vi "Teleop.vi"(10 "Match Info":T1={"Autonomous Elapsed Seconds"=0.0, "TeleOp Elapsed Seconds"=0.0, "Disabled Elapsed Seconds"=0.0, "Visited Autonomous"=FALSE, "Visited TeleOp"=FALSE, "Visited Disabled"=FALSE, "Autonomous Settings"={"Autonomous Style"=enum."Independent", "VI Refnum"=refnum}}, 11 "Call Context":T2) -> ()   [LabVIEW 2015]
doc: "This VI is called for each TeleOp packet received from the DS where the robot is not disabled. It is often used to read from the joysticks and update I/O or to update setpoints for timed control loops. It should complete and return within 20 milliseconds or it may miss DS packets."
uses:
  <vilib>/Rock Robotics/WPI/DriverStation/WPI_DriverStationDerivedRobotMode.ctl
  <vilib>/Rock Robotics/WPI/DriverStation/WPI_DriverStationMatch Info.ctl
  <vilib>/Rock Robotics/WPI/Utilities/WPI_GetSetVariantRefNum.vi
  <vilib>/Rock Robotics/Network Tables/NT Write Boolean Array.vi
  <vilib>/Rock Robotics/Network Tables/NT Write Numeric Array.vi
  <vilib>/Rock Robotics/Network Tables/NT Read Boolean.vi
  <vilib>/Rock Robotics/Network Tables/NT Read Number.vi
  <vilib>/Rock Robotics/Network Tables/NT Write Number.vi
  <vilib>/Rock Robotics/Network Tables/NT Write Boolean.vi
panel:
  out "Sample Slider 0":dbl(slide) scale=0.0..5.0
  out "Sample Boolean 1":bool
  out "Sample Boolean 0":bool
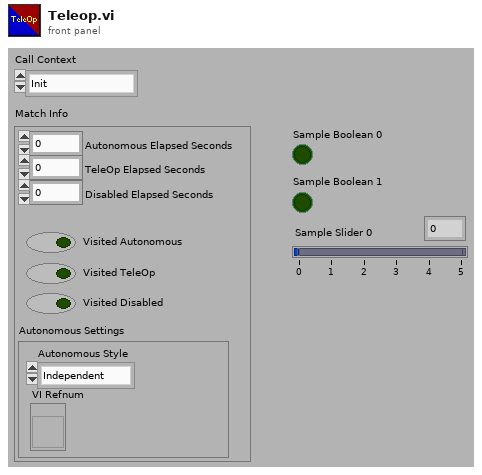
[diagram p1: front panel]
types:
  T1 = typedef "WPI_DriverStationMatch Info.ctl" = cluster{"Autonomous Elapsed Seconds":dbl, "TeleOp Elapsed Seconds":dbl, "Disabled Elapsed Seconds":dbl, "Visited Autonomous":bool, "Visited TeleOp":bool, "Visited Disabled":bool, "Autonomous Settings":cluster{"Autonomous Style":enum16{"Iterative", "Independent"}, "VI Refnum":refnum<vi>}}
  T2 = typedef "WPI_DriverStationDerivedRobotMode.ctl" = enum16{"Init", "Execute", "Stop"}
  T3 = typedef "WPI_MotorControlDeviceRef.ctl" = cluster{"DeviceStatus":errorcluster, "Type":T4, "PWM":cluster{"PWM Channel":T5, "DeadBand":T6}, "CAN":cluster{"Device Number":u8, "Control Mode":T7, "Semaphore":T8, "Max Vout":dbl, "TalonSRX Control Mode":T9}, "Invert":bool}
  T4 = typedef "WPI_MotorControlType.ctl" = enum16{"PWM", "CAN", "CANTalonSRX"}
  T5 = typedef "FPGA_DIOPWMChannel.ctl" = enum8{"PWM 0", "PWM 1", "PWM 2", "PWM 3", "PWM 4", "PWM 5", "PWM 6", "PWM 7", "PWM 8", "PWM 9", "PWM MXP 0", "PWM MXP 1", "PWM MXP 2", "PWM MXP 3", "PWM MXP 4", "PWM MXP 5", "PWM MXP 6", "PWM MXP 7", "PWM MXP 8", "PWM MXP 9", "Invalid"}
  T6 = typedef "WPI_PWMDeadband.ctl" = cluster{"Name":string, "maxPositivePwm":i32, "minPositivePwm":i32, "centerPwm":i32, "maxNegativePwm":i32, "minNegativePwm":i32, "angularRange":u16}
  T7 = typedef "WPI_CANJaguar_ControlMode.ctl" = enum8{"Percent VBus", "Current", "Speed", "Position", "Voltage"}
  T8 = typedef "Semaphore RefNum" = refnum<k1>
  T9 = typedef "WPI_CANTalonSRX_APIControlMode.ctl" = enum8{"Percent VBus", "Speed", "Position", "Slave", "Unchanged / Invalid", "Voltage Compensation", "Current", "Motion Profile"}
  T10 = typedef "WPI_RobotDriveDevRef.ctl" = cluster{"DevStatus":errorcluster, "Motors[]":T3[], "Square Inputs":bool, "Max Output":dbl}
  T11 = typedef "WPI_JoystickDevRef.ctl" = cluster{"Device":T12}
  T12 = typedef "WPI_JoystickDeviceEnum.ctl" = enum16{"USB 0", "USB 1", "USB 2", "USB 3", "USB 4", "USB 5"}
  T13 = typedef "WPI_DigitalInputDevRef.ctl" = cluster{"DevStatus":errorcluster, "DIO Channel":T14}
  T14 = typedef "FPGA_DIOChannel.ctl" = enum8{"DIO 0", "DIO 1", "DIO 2", "DIO 3", "DIO 4", "DIO 5", "DIO 6", "DIO 7", "DIO 8", "DIO 9", "DIO MXP 0", "DIO MXP 1", "DIO MXP 2", "DIO MXP 3", "DIO MXP 4", "DIO MXP 5", "DIO MXP 6", "DIO MXP 7", "DIO MXP 8", "DIO MXP 9", "DIO MXP 10", "DIO MXP 11", "DIO MXP 12", "DIO MXP 13", "DIO MXP 14", "DIO MXP 15", "Invalid"}
  T15 = typedef "WPI_ServoDeviceRef.ctl" = cluster{"DeviceStatus":errorcluster, "PWM Channel":T5, "DeadBand":T6}
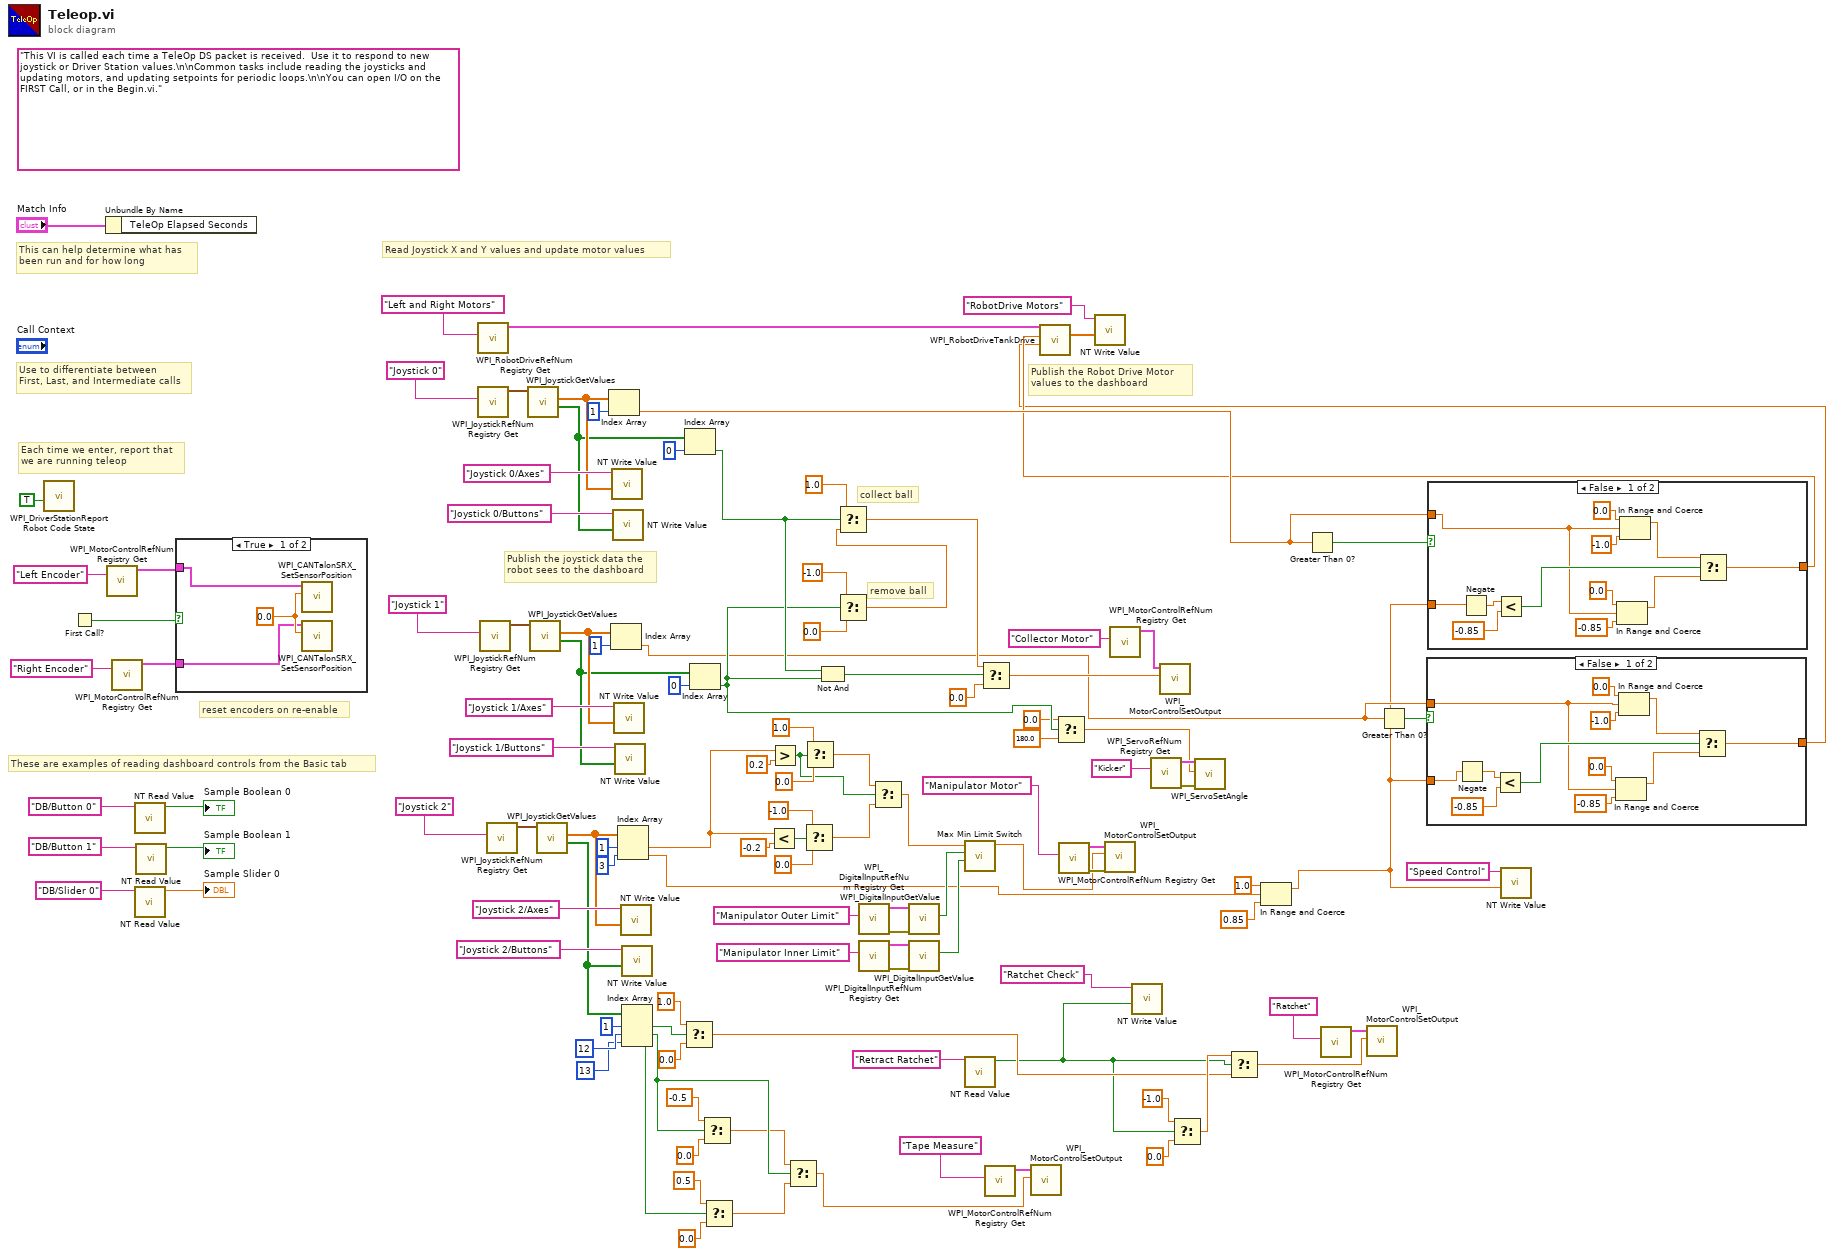
[diagram p0: block diagram]
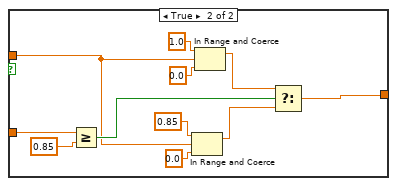
[diagram p2: hidden frame]
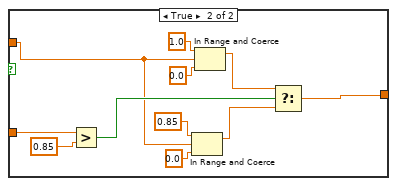
[diagram p3: hidden frame]
diagram:
  (unwired) "This VI is called each time a TeleOp DS packet is received.  Use it to respond to new joystick or Driver Station values.\n\nCommon tasks include reading the joysticks and updating motors, and updating setpoints for periodic loops.\n\nYou can open I/O on the FIRST Call, or in the Begin.vi."
  # "remove ball"
  # "collect ball"
  # "reset encoders on re-enable"
  # "These are examples of reading dashboard controls from the Basic tab"
  # "Publish the Robot Drive Motor\nvalues to the dashboard"
  # "Publish the joystick data the\nrobot sees to the dashboard"
  # "Each time we enter, report that\nwe are running teleop"
  # "Use to differentiate between\nFirst, Last, and Intermediate calls"
  # "This can help determine what has\nbeen run and for how long"
  # "Read Joystick X and Y values and update motor values"
  n1 = call <vilib>:"WPI_DriverStationReport Robot Code State.vi"("TeleOp"=TRUE ("Autonomous")) -> ()  [unwired: 10 in, 1 out]
  n2 = First Call?() -> (First Call?: T/F=w104:bool)
  n3 = Unbundle By Name("Match Info") -> ()  [unwired: 1 out]
  n4 = call <vilib>:"WPI_MotorControlRefNum Registry Get.vi"("refnum name"="Left Encoder") -> ("MotorControlDevRef"=w102:T3)  [unwired: 9 in, 1 out]
  n5 = call <vilib>:"WPI_MotorControlRefNum Registry Get.vi"("refnum name"="Right Encoder") -> ("MotorControlDevRef"=w101:T3)  [unwired: 9 in, 1 out]
  n6 = call-poly <vilib>:"NT Read Value.vi"("Name"="DB/Button 0" ("refnum name")) -> ("Boolean"=→"Sample Boolean 0":bool)  [unwired: 9 in, 1 out]
  n7 = call-poly <vilib>:"NT Read Value.vi"("Name"="DB/Slider 0" ("refnum name")) -> ("Numeric"=→"Sample Slider 0":dbl)  [unwired: 9 in, 1 out]
  n8 = call-poly <vilib>:"NT Read Value.vi"("Name"="DB/Button 1" ("refnum name")) -> ("Boolean"=→"Sample Boolean 1":bool)  [unwired: 9 in, 1 out]
  n9 = case shown="True" w104 {
    tunnel: w102 -> [w123 _]
    tunnel: w101 -> [w122 _]
    frame True {
      w124 = 0.0
      n10 = call <vilib>:"WPI_CANTalonSRX_SetSensorPosition.vi"("New Sensor Position"=w124, "CAN Talon SRX Ref"=w123) -> ()  [unwired: 8 in, 2 out]
      n11 = call <vilib>:"WPI_CANTalonSRX_SetSensorPosition.vi"("New Sensor Position"=w124, "CAN Talon SRX Ref"=w122) -> ()  [unwired: 8 in, 2 out]
    }
    frame False {
    }
  }
  n12 = call <vilib>:"WPI_RobotDriveRefNum Registry Get.vi"("refnum name"="Left and Right Motors") -> ("RobotDriveDevRef"=w119:T10)  [unwired: 1 in, 9 out]
  n13 = call <vilib>:"WPI_JoystickRefNum Registry Get.vi"("refnum name"="Joystick 0") -> ("JoystickDevRef"=w117:T11)  [unwired: 1 in, 9 out]
  n14 = call <vilib>:"WPI_JoystickRefNum Registry Get.vi"("refnum name"="Joystick 1") -> ("JoystickDevRef"=w99:T11)  [unwired: 1 in, 9 out]
  n15 = call <vilib>:"WPI_JoystickRefNum Registry Get.vi"("refnum name"="Joystick 2") -> ("JoystickDevRef"=w92:T11)  [unwired: 1 in, 9 out]
  n16 = call <vilib>:"WPI_JoystickGetValues.vi"("JoystickDevRef"=w117) -> ("Buttons"=w78:bool[], "Axes"=w113:dbl[])  [unwired: 6 in, 3 out]
  n17 = call <vilib>:"WPI_JoystickGetValues.vi"("JoystickDevRef"=w99) -> ("Buttons"=w87:bool[], "Axes"=w96:dbl[])  [unwired: 6 in, 3 out]
  n18 = call <vilib>:"WPI_JoystickGetValues.vi"("JoystickDevRef"=w92) -> ("Buttons"=w28:bool[], "Axes"=w89:dbl[])  [unwired: 6 in, 3 out]
  n19 = Index Array(array=w113, index=1) -> (element=w36:dbl)
  n20 = Index Array(array=w96, index=1) -> (element=w35:dbl)
  n21 = call-poly <vilib>:"NT Write Value.vi"("Numeric Array"=w113, "Name"="Joystick 0/Axes") -> ()  [unwired: 9 in, 1 out]
  n22 = call-poly <vilib>:"NT Write Value.vi"("Boolean Array"=w78, "Name"="Joystick 0/Buttons") -> ()  [unwired: 9 in, 1 out]
  n23 = call-poly <vilib>:"NT Write Value.vi"("Numeric Array"=w96, "Name"="Joystick 1/Axes") -> ()  [unwired: 9 in, 1 out]
  n24 = call-poly <vilib>:"NT Write Value.vi"("Boolean Array"=w87, "Name"="Joystick 1/Buttons") -> ()  [unwired: 9 in, 1 out]
  n25 = Index Array(array=w89, index #1=1 ("index"), index #2=3 ("index")) -> (element #1=w53:dbl, element #2=w30:dbl)
  n26 = call-poly <vilib>:"NT Write Value.vi"("Numeric Array"=w89, "Name"="Joystick 2/Axes") -> ()  [unwired: 9 in, 1 out]
  n27 = call-poly <vilib>:"NT Write Value.vi"("Boolean Array"=w28, "Name"="Joystick 2/Buttons") -> ()  [unwired: 9 in, 1 out]
  n28 = Index Array(array=w28, index #1=1 ("index"), index #2=12 ("index"), index #3=13 ("index")) -> (element #1=w25:bool, element #2=w12:bool, element #3=w15:bool)
  n29 = Select(t=1.0, s=w25, f=0.0) -> (s? t:f=w3:dbl)
  n30 = Index Array(array=w78, index=0) -> (element=w76:bool)
  n31 = Index Array(array=w87, index=0) -> (element=w44:bool)
  n32 = Select(t=-0.5, s=w12, f=0.0) -> (s? t:f=w11:dbl)
  n33 = Select(t=0.5, s=w15, f=0.0) -> (s? t:f=w10:dbl)
  n34 = Less?(x=w53, y=-0.2) -> (x < y?=w56:bool)
  n35 = Greater?(x=w53, y=0.2) -> (0:w52:bool)
  n36 = Select(t=w11, s=w12, f=w10) -> (s? t:f=w9:dbl)
  n37 = Select(t=-1.0, s=w56, f=0.0) -> (s? t:f=w50:dbl)
  n38 = Select(t=1.0, s=w52, f=0.0) -> (s? t:f=w51:dbl)
  n39 = Not And(1:w44, 2:w76) -> (0:w81:bool)
  n40 = Select(t=-1.0, s=w44, f=0.0) -> (s? t:f=w82:dbl)
  n41 = Select(t=1.0, s=w76, f=w82) -> (s? t:f=w79:dbl)
  n42 = call <vilib>:"WPI_DigitalInputRefNum Registry Get.vi"("refnum name"="Manipulator Outer Limit") -> ("error out"=w72:errorcluster, "DigitalInputDevRef"=w71:T13)  [unwired: 9 in]
  n43 = call <vilib>:"WPI_DigitalInputRefNum Registry Get.vi"("refnum name"="Manipulator Inner Limit") -> ("error out"=w70:errorcluster, "DigitalInputDevRef"=w69:T13)  [unwired: 9 in]
  n44 = Select(t=w51, s=w52, f=w50) -> (s? t:f=w49:dbl)
  n45 = call <vilib>:"WPI_DigitalInputGetValue.vi"("error in (no error)"=w72, "DigitalInputDevRef"=w71) -> ("Value"=w62:bool)  [unwired: 7 in, 2 out]
  n46 = call <vilib>:"WPI_DigitalInputGetValue.vi"("error in (no error)"=w70, "DigitalInputDevRef"=w69) -> ("Value"=w61:bool)  [unwired: 7 in, 2 out]
  n47 = call "Max Min Limit Switch.vi"("Lower Limit"=w61, "Upper Limit"=w62, "Input"=w49) -> ("Output"=w48:dbl)  [unwired: 8 in]
  n48 = call-poly <vilib>:"NT Read Value.vi"("Name"="Retract Ratchet") -> ("Boolean"=w2:bool)  [unwired: 9 in, 1 out]
  n49 = Select(t=w79, s=w81, f=0.0) -> (s? t:f=w74:dbl)
  n50 = call <vilib>:"WPI_MotorControlRefNum Registry Get.vi"("refnum name"="Tape Measure") -> ("MotorControlDevRef"=w14:T3)  [unwired: 9 in, 1 out]
  n51 = call <vilib>:"WPI_MotorControlSetOutput.vi"("Output"=w9, "MotorControlDevRef"=w14) -> ()  [unwired: 7 in, 3 out]
  n52 = Select(t=0.0, s=w44, f=180.0) -> (s? t:f=w43:dbl)
  n53 = call <vilib>:"WPI_MotorControlRefNum Registry Get.vi"("refnum name"="Manipulator Motor") -> ("error out"=w66:errorcluster, "MotorControlDevRef"=w65:T3)  [unwired: 9 in]
  n54 = call <vilib>:"WPI_MotorControlSetOutput.vi"("error in (no error)"=w66, "Output"=w48, "MotorControlDevRef"=w65) -> ()  [unwired: 6 in, 3 out]
  n55 = call <vilib>:"WPI_MotorControlRefNum Registry Get.vi"("refnum name"="Collector Motor") -> ("MotorControlDevRef"=w73:T3)  [unwired: 9 in, 1 out]
  n56 = call-poly <vilib>:"NT Write Value.vi"("Boolean"=w2, "Name"="Ratchet Check") -> ()  [unwired: 9 in, 1 out]
  n57 = call <vilib>:"WPI_ServoRefNum Registry Get.vi"("refnum name"="Kicker") -> ("error out"=w46:errorcluster, "ServoDeviceRef"=w45:T15)  [unwired: 9 in]
  n58 = call <vilib>:"WPI_MotorControlSetOutput.vi"("Output"=w74, "MotorControlDevRef"=w73) -> ()  [unwired: 7 in, 3 out]
  n59 = Select(t=-1.0, s=w2, f=0.0) -> (s? t:f=w4:dbl)
  n60 = call <vilib>:"WPI_ServoSetAngle.vi"("error in (no error)"=w46, "Angle"=w43, "ServoDeviceRef"=w45) -> ()  [unwired: 7 in, 2 out]
  n61 = Select(t=w4, s=w2, f=w3) -> (s? t:f=w7:dbl)
  n62 = In Range and Coerce(upper limit=1.0, x=w30, lower limit=0.85) -> (coerced(x)=w32:dbl)  [unwired: 1 out]
  n63 = Greater Than 0?(x=w36) -> (x > 0?=w38:bool)
  n64 = call <vilib>:"WPI_MotorControlRefNum Registry Get.vi"("refnum name"="Ratchet") -> ("MotorControlDevRef"=w26:T3)  [unwired: 9 in, 1 out]
  n65 = call <vilib>:"WPI_MotorControlSetOutput.vi"("Output"=w7, "MotorControlDevRef"=w26) -> ()  [unwired: 7 in, 3 out]
  n66 = Greater Than 0?(x=w35) -> (x > 0?=w37:bool)
  n67 = case shown="False" w37 {
    tunnel: w32 -> [w126 w146]
    tunnel: [w128 w138] -> w33
    tunnel: w35 -> [w125 w137]
    frame False {
      n68 = Negate(x=w126) -> (-x=w127:dbl)
      n69 = Less?(x=w127, y=-0.85) -> (x < y?=w129:bool)
      n70 = In Range and Coerce(upper limit=0.0, x=w125, lower limit=-0.85) -> (coerced(x)=w130:dbl)  [unwired: 1 out]
      n71 = In Range and Coerce(upper limit=0.0, x=w125, lower limit=-1.0) -> (coerced(x)=w135:dbl)  [unwired: 1 out]
      n72 = Select(t=w135, s=w129, f=w130) -> (s? t:f=w128:dbl)
    }
    frame True {
      n73 = Greater Or Equal?(x=w146, y=0.85) -> (x >= y?=w139:bool)
      n74 = In Range and Coerce(upper limit=0.85, x=w137, lower limit=0.0) -> (coerced(x)=w140:dbl)  [unwired: 1 out]
      n75 = In Range and Coerce(upper limit=1.0, x=w137, lower limit=0.0) -> (coerced(x)=w145:dbl)  [unwired: 1 out]
      n76 = Select(t=w145, s=w139, f=w140) -> (s? t:f=w138:dbl)
    }
  }
  n77 = case shown="False" w38 {
    tunnel: w32 -> [w150 w169]
    tunnel: [w151 w161] -> w34
    tunnel: w36 -> [w148 w160]
    frame False {
      n78 = Negate(x=w150) -> (-x=w149:dbl)
      n79 = Less?(x=w149, y=-0.85) -> (x < y?=w152:bool)
      n80 = In Range and Coerce(upper limit=0.0, x=w148, lower limit=-0.85) -> (coerced(x)=w153:dbl)  [unwired: 1 out]
      n81 = In Range and Coerce(upper limit=0.0, x=w148, lower limit=-1.0) -> (coerced(x)=w158:dbl)  [unwired: 1 out]
      n82 = Select(t=w158, s=w152, f=w153) -> (s? t:f=w151:dbl)
    }
    frame True {
      n83 = Greater?(x=w169, y=0.85) -> (0:w162:bool)
      n84 = In Range and Coerce(upper limit=0.85, x=w160, lower limit=0.0) -> (coerced(x)=w163:dbl)  [unwired: 1 out]
      n85 = In Range and Coerce(upper limit=1.0, x=w160, lower limit=0.0) -> (coerced(x)=w168:dbl)  [unwired: 1 out]
      n86 = Select(t=w168, s=w162, f=w163) -> (s? t:f=w161:dbl)
    }
  }
  n87 = call <vilib>:"WPI_RobotDriveTankDrive.vi"("Right axis value"=w33, "Left axis value"=w34, "RobotDriveDevRef"=w119) -> ("Motor Values"=w106:dbl[])  [unwired: 6 in, 2 out]
  n88 = call-poly <vilib>:"NT Write Value.vi"("Numeric Array"=w106, "Name"="RobotDrive Motors") -> ()  [unwired: 9 in, 1 out]
  n89 = call-poly <vilib>:"NT Write Value.vi"("Numeric"=w32, "Name"="Speed Control") -> ()  [unwired: 9 in, 1 out]
